vi "report.bin to bin result test.vi"(7 "Result test":bool, 13 "Test?":bool) -> (8 "T= T test or No data":bool)   [LabVIEW 2019]
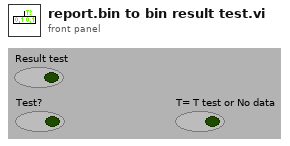
[diagram p1: front panel]
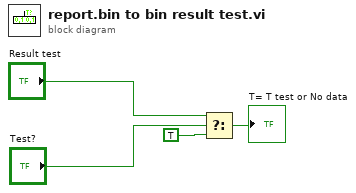
[diagram p0: block diagram]
diagram:
  n1 = Select(t="Result test", s="Test?", f=TRUE) -> (s? t:f=→"T= T test or No data":bool)
